vi "setWaveformType.vi"(8 "error in (no error)":errorcluster, 10 "Waveform":enum16{"Sine", "Rectangular", "Triangular"}(ring), 11 "VISA resource name":refnum<visa-resource-name>) -> (0 "error out":errorcluster, 3 "VISA resource name out":refnum<visa-resource-name>)   [LabVIEW 2023, in "Keysight-33500B.lvlib"]
doc: "<b>Author:</b> Wolfgang Rominger\n<b>Description:</b> >>>> VI configuring the AWG to the selected waveforms >>>"
uses:
  Keysight-33500B.lvlib
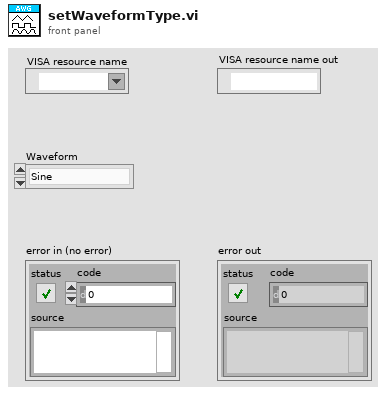
[diagram p1: front panel]
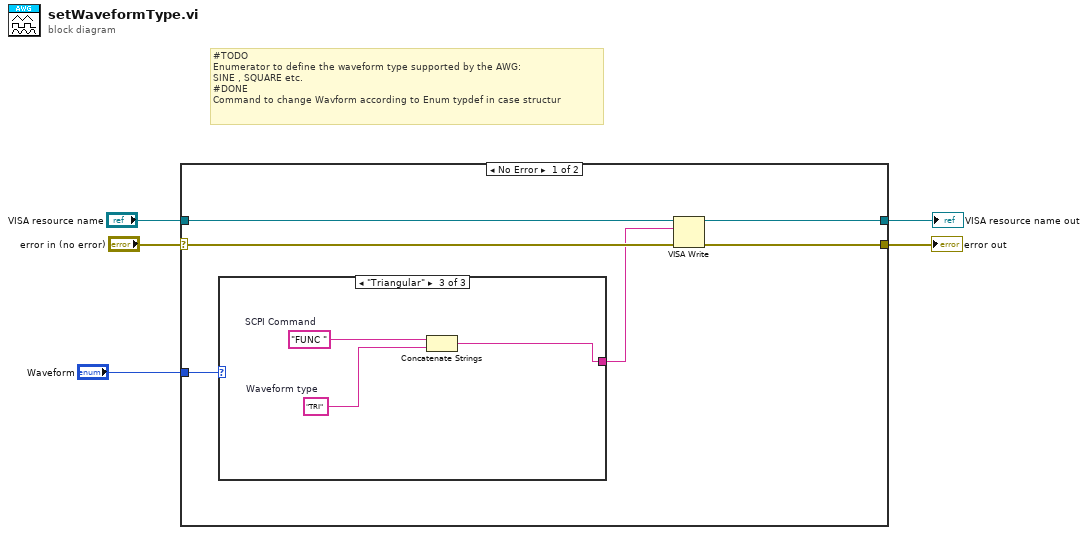
[diagram p0: block diagram]
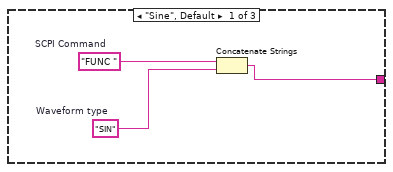
[diagram p2: hidden frame]
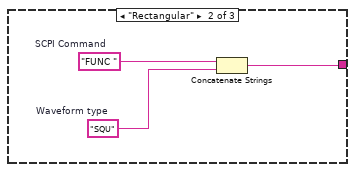
[diagram p3: hidden frame]
diagram:
  # "#TODO\nEnumerator to define the waveform type supported by the AWG:\nSINE , SQUARE etc.\n#DONE\nCommand to change Wavform according to Enum typdef in case structur"
  n1 = case shown="No Error" "error in (no error)" {
    selector: "error in (no error)" -> [w8 w22]
    tunnel: [w10 w21] -> w5
    tunnel: [w11 w22] -> w3
    tunnel: "VISA resource name" -> [w9 w21]
    tunnel: "Waveform" -> [w7 _]
    frame No Error {
      n2 = case shown="\"Triangular\"" w7 {
        tunnel: [w12 w15 w18] -> w6
        frame "Sine", Default {
          w13 = "SIN"  # Waveform type
          w14 = "FUNC "  # SCPI Command
          n3 = Concatenate Strings(w14, w13) -> (w12:string)
        }
        frame "Rectangular" {
          w16 = "SQU"  # Waveform type
          w17 = "FUNC "  # SCPI Command
          n4 = Concatenate Strings(w17, w16) -> (w15:string)
        }
        frame "Triangular" {
          w19 = "TRI"  # Waveform type
          w20 = "FUNC "  # SCPI Command
          n5 = Concatenate Strings(w20, w19) -> (w18:string)
        }
      }
      n6 = VISA Write(VISA resource name=w9, write buffer=w6, error in (no error)=w8) -> (VISA resource name out=w10:refnum<visa-resource-name>, error out=w11:errorcluster)  [unwired: 1 out]
    }
    frame Error {
    }
  }
  "VISA resource name out" <- w5
  "error out" <- w3
